vi "Place actuators to the Home Positions.vi"(8 "error in":errorcluster, 10 "Time to wait":i32=999, 11 "UTP IO Session in":T1) -> (0 "error out":errorcluster, 2 "ExpiredTimeToWait?":bool, 3 "UTP IO Session out":T1)   [LabVIEW 2023, in "Actuators.lvlib"]
doc: "Sending all of the actuators to their Home Position\nPeriod for reading is 10ms"
uses:
  Actuators.lvlib
  <vilib>/Noffz/UTP IO/UTP IO Library/Typedefs/Session Handle.ctl
  <vilib>/Noffz/UTP IO/UTP IO Library/UTP IO Pool Session.lvclass
  <vilib>/Noffz/UTP IO/UTP IO Library/methods/poly/plc/Write PLC Variable (Boolean).vi
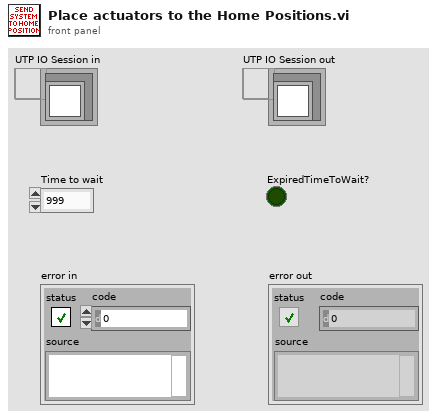
[diagram p1: front panel]
types:
  T1 = typedef "UTP IO Library.lvlib/UTP IO Pool Session.lvclass/Session Handle.ctl" = refnum<data-value>
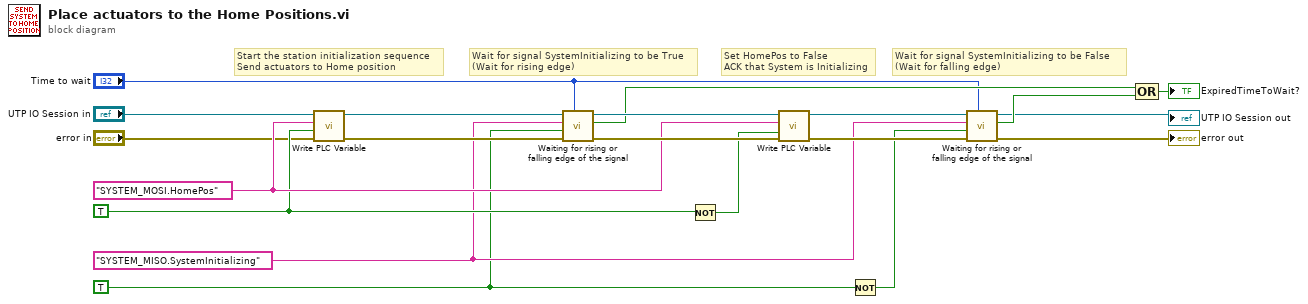
[diagram p0: block diagram]
diagram:
  w9 = TRUE ("Rising/Falling edge")
  w10 = "SYSTEM_MISO.SystemInitializing" ("variable name")
  w14 = TRUE ("value")
  w15 = "SYSTEM_MOSI.HomePos" ("variable name")
  # "Wait for signal SystemInitializing to be False \n(Wait for falling edge)"
  # "Wait for signal SystemInitializing to be True\n(Wait for rising edge)"
  # "Set HomePos to False \nACK that System is Initializing"
  # "Start the station initialization sequence \nSend actuators to Home position"
  n1 = call-poly <vilib>:"Write PLC Variable.vi"("error in (no error)"="error in", "value"=w14, "variable name"=w15, "UTP IO Session in"="UTP IO Session in") -> ("error out"=w18:errorcluster, "UTP IO Session out"=w19:T1)  [unwired: 6 in]
  n2 = call "Waiting for rising or falling edge of the signal.vi"("Time to wait"="Time to wait", "error in"=w18, "Rising/Falling edge"=w9, "Variable name"=w10, "UTP IO Session in"=w19) -> ("error out"=w16:errorcluster, "ExpiredTimeToWait?"=w5:bool, "UTP IO Session out"=w17:T1)  [unwired: 4 in]
  n3 = Not(x=w14) -> (.not. x?=w13:bool)
  n4 = call-poly <vilib>:"Write PLC Variable.vi"("error in (no error)"=w16, "value"=w13, "variable name"=w15, "UTP IO Session in"=w17) -> ("error out"=w11:errorcluster, "UTP IO Session out"=w12:T1)  [unwired: 6 in]
  n5 = Not(x=w9) -> (.not. x?=w8:bool)
  n6 = call "Waiting for rising or falling edge of the signal.vi"("Time to wait"="Time to wait", "error in"=w11, "Rising/Falling edge"=w8, "Variable name"=w10, "UTP IO Session in"=w12) -> ("error out"=→"error out":errorcluster, "ExpiredTimeToWait?"=w6:bool, "UTP IO Session out"=→"UTP IO Session out":T1)  [unwired: 4 in]
  n7 = Compound Arithmetic op=OR(w5, w6) -> (→"ExpiredTimeToWait?":bool)
